vi "mask_circular.vi"(8 "clu_mask_cor":T1, 11 "image in":T2) -> (0 "u8_ar_mask":u8[][](array[numeric]), 3 "masekd image out":T2)   [LabVIEW 2011]
uses:
  <vilib>/vision/Image Controls.llb/IMAQ Image.ctl
  <vilib>/vision/NI_Vision_Development_Module.lvlib
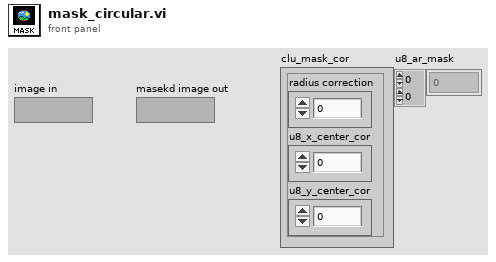
[diagram p1: front panel]
types:
  T1 = cluster{"radius correction":i16, "u8_x_center_cor":i16, "u8_y_center_cor":i16}
  T2 = typedef "IMAQ Image.ctl" = refnum<image>
  T3 = typedef "IMAQ Circle" = cluster{"Center X":i32, "Center Y":i32, "Inner Radius":i32, "Outer Radius":i32, "Start Angle":dbl, "End Angle":dbl}
  T4 = typedef "Image Type" = u32
  T5 = typedef "ROI Descriptor" = cluster{"Global Rectangle":i32[], "Contours":cluster{"ID":enum32{"External", "Internal"}, "Type":u32, "Coordinates":i32[]}[]}
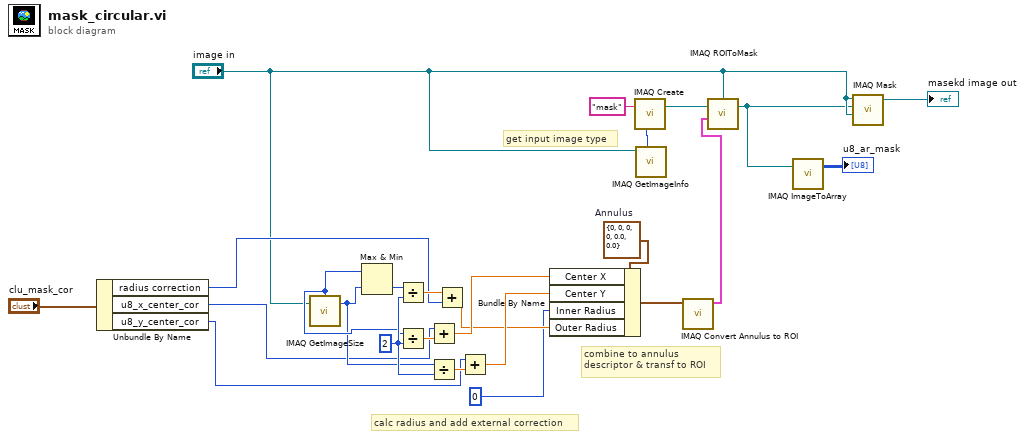
[diagram p0: block diagram]
diagram:
  w18 = T3 {"Center X"=0, "Center Y"=0, "Inner Radius"=0, "Outer Radius"=0, "Start Angle"=0.0, "End Angle"=0.0}  # Annulus
  w21 = 2 ("y")
  # "get input image type"
  # "combine to annulus\ndescriptor & transf to ROI"
  # "calc radius and add external correction"
  n1 = Unbundle By Name("clu_mask_cor") -> ("radius correction"=w9:i16, "u8_x_center_cor"=w8:i16, "u8_y_center_cor"=w7:i16)
  n2 = call "IMAQ GetImageSize"("Image"="image in") -> ("Y Resolution"=w16:i32, "X Resolution"=w17:i32)  [unwired: 3 in, 1 out]
  n3 = Max & Min(x=w17, y=w16) -> (min(x,y)=w20:i32)  [unwired: 1 out]
  n4 = Divide(x=w20, y=w21) -> (x/y=w22:dbl)
  n5 = Divide(x=w17, y=w21) -> (x/y=w13:dbl)
  n6 = Add(x=w8, y=w13) -> (x+y=w25:dbl)
  n7 = Divide(x=w16, y=w21) -> (x/y=w14:dbl)
  n8 = Add(x=w22, y=w9) -> (x+y=w23:dbl)
  n9 = Add(x=w7, y=w14) -> (x+y=w24:dbl)
  n10 = Bundle By Name(cluster=w18, "Center X"=w25, "Center Y"=w24, "Inner Radius"=0, "Outer Radius"=w23) -> (w19:T3)
  n11 = call "IMAQ GetImageInfo"("Image"="image in") -> ("Image Type"=w3:T4)  [unwired: 3 in, 7 out]
  n12 = call "IMAQ Create"("Image Name"="mask", "Image Type"=w3) -> ("New Image"=w5:T2)  [unwired: 3 in, 1 out]
  n13 = call "IMAQ Convert Annulus to ROI"("Annulus"=w19) -> ("ROI Descriptor"=w12:T5)  [unwired: 8 in, 1 out]
  n14 = call "IMAQ ROIToMask"("ROI Descriptor"=w12, "Image"=w5, "Image Model"="image in") -> ("Image Out"=w2:T2)  [unwired: 2 in, 3 out]
  n15 = call "IMAQ ImageToArray"("Image"=w2) -> ("Image Pixels (U8)"=→"u8_ar_mask":u8[][])  [unwired: 3 in, 4 out]
  n16 = call "IMAQ Mask"("Image Dst"="image in", "Image Mask"=w2, "Image Src"="image in") -> ("Image Dst Out"=→"masekd image out":T2)  [unwired: 2 in, 1 out]
